vi "SaveImages_Example.vi"() -> ()   [LabVIEW 2019]
doc: "This example shows how to record an image sequence and save all images to files (and an .avi) afterwards.\nIt is a good starting point for writing own applications with file saving\nBut it will not be fail save, i.e. doesnt react on errors, just handles them forward to the end\n\nUsage:\nSelect your required image count you want to record before you start the program.\nOnce started, the camera class will be initialized and images will be recorded automatically.\nWhen acquisition has finished you can read the images by index, crop them using the ROI parameters and select a file path.\nBy clicking save, the images are saved with the selected file format using the current active roi setting.\nThis also finishes the program and will force an exit of the camera class"
uses:
  camera/Camera.lvclass
  pco.recorder/Recorder.lvlib
  <vilib>/picture/picture.llb/Draw 8-Bit Pixmap.vi
  <vilib>/picture/picture.llb/Draw True-Color Pixmap.vi
panel:
  out "colormap(U8)":u32[](array[numeric])
  out "Image(U16)":u16[][](graph)
  in  "Zoom [%]":i32(slide)=26 min=10 max=200 step=5 scale=10.0..200.0
  out "Image":picture
  out "rawImage":u16[][](array[numeric])
  in  "data_format":T1(ring)=enum."Mono16"
  in  "Image Index":u32 max=9
  in  "saveImages":bool
  in  "SavePath":path
  out "Recorded Images":u32
  in  "Quit":bool
  in  "cropY1":u64=2 min=2 max=2048 step=1
  in  "cropX1":u64=2 min=2 max=2048 step=1
  in  "cropY0":u64=1 min=1 max=2047 step=1
  in  "cropX0":u64=1 min=1 max=2047 step=1
  out "Image Height":u16
  out "Image Width":u16
  in  "dwImgCount":u32=10 caption="Required Number of Images" max=4023
  out "Error":errorcluster {"code" format="%x"}
  # "This example shows how to record an image sequence and save all images to files (and an .avi) afterwards.\nIt is a good starting point for writing own applications with file saving\nBut it will not be fail save, i.e. doesnt react on errors, just handles them forward to the end\n\nUsage:\nSelect your required image count you want to record before you start the program.\nOnce started, the camera class will be initialized and images will be recorded automatically.\nWhen acquisition has finished you can read the images by index, crop them using the crop parameters and select a file path.\nBy clicking save, the images are saved with the selected file format using the current active roi setting.\nThis also finishes the program and will force an exit of the camera class"
  # "pco.labview"
  # "Camera Setup"
  # "Recording Control"
  # "Parameters for image readout"
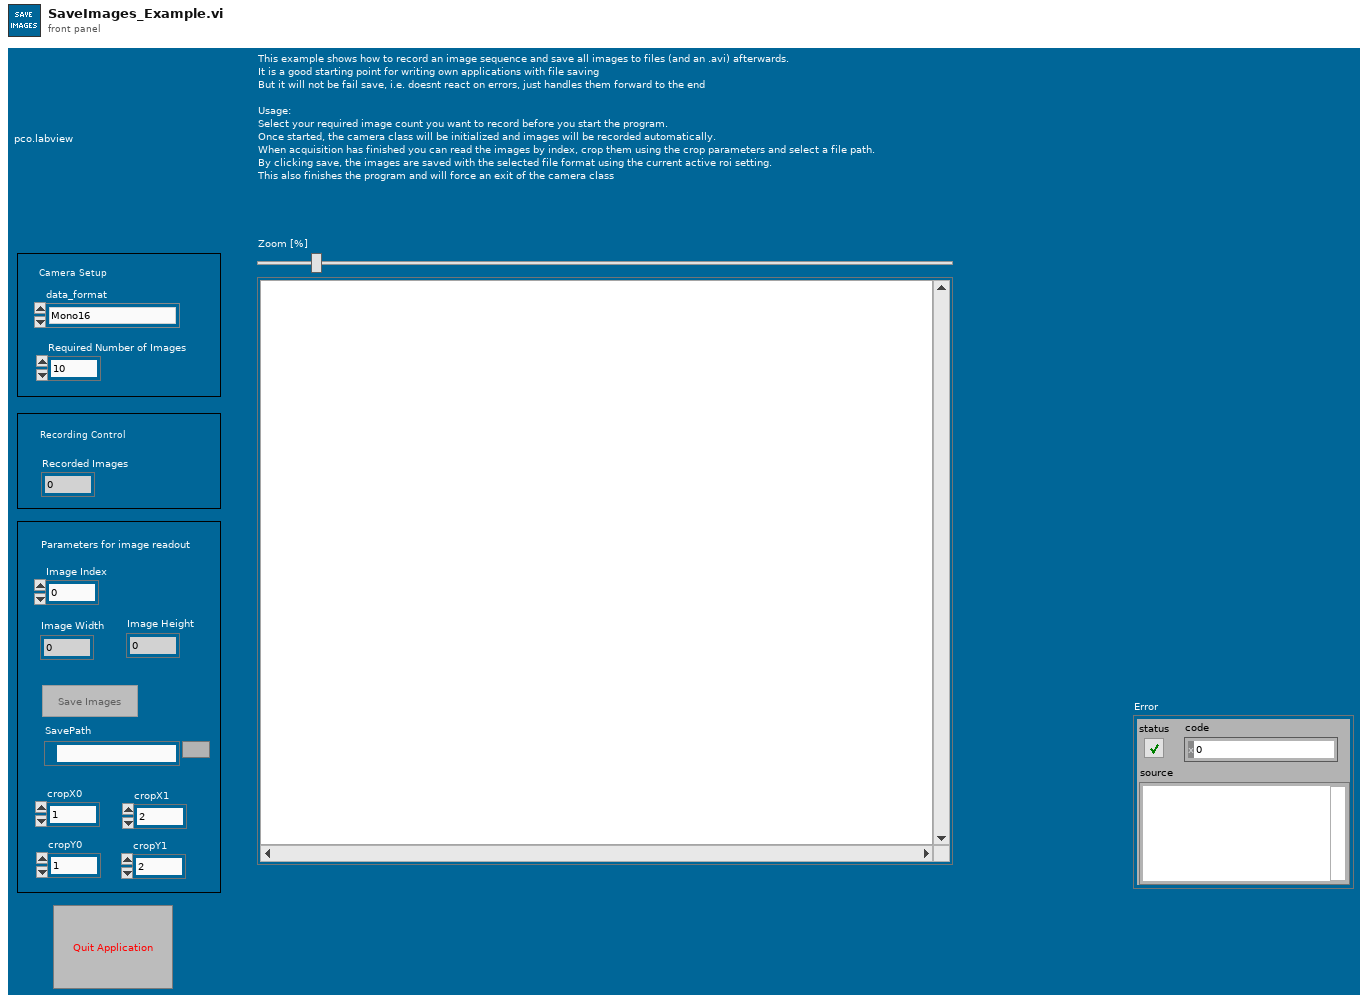
[diagram p1: front panel]
types:
  T1 = enum16{"Undefined", "Mono8", "Mono16", "BGRA8", "RGBA8", "BGRA16", "RGBA16", "CompressedMono8"}
  T2 = enum8{"Enabled", "Disabled", "Disabled and Grayed Out"}
  T3 = enum16{"sequence", "sequence non blocking", "ring buffer", "fifo", "tif", "multitif", "pcoraw", "b16", "dicom", "multidicom", "camram_ring", "camram_segment"}
  T4 = typedef "Camera.lvclass/binning.ctl" = cluster{"vert":u16, "horz":u16, "mode":u16}
  T5 = cluster{"exposure_time_s":dbl, "delay_time_s":dbl, "roi":cluster{"x0":u64, "y0":u64, "x1":u64, "y1":u64}, "timestamp_mode":u16, "pixelrate":u32, "conversion_factor":sgl, "trigger_mode":u16, "acquire_mode":u16, "acquire_sequence_number":u32, "metadata_mode":u16, "noisefilter_mode":u16, "pixel_format":u32, "binning":T4, "auto_exposure":cluster{"region":u16, "min_exposure_s":dbl, "max_exposure_s":dbl}}
  T6 = cluster{"wVersion":u16, "dwIMAGE_COUNTER":u32, "dwIMAGE_TIME_US":u32, "lvTimestamp":timestamp, "bIMAGE_TIME_STATUS":u8, "wEXPOSURE_TIME_BASE":u16, "dwEXPOSURE_TIME":u32, "dwFRAMERATE_MILLIHZ":u32, "sSENSOR_TEMPERATURE":i16, "wIMAGE_SIZE_X":u16, "wIMAGE_SIZE_Y":u16, "bBINNING_X":u8, "bBINNING_Y":u8, "dwSENSOR_READOUT_FREQUENCY":u32, "wSENSOR_CONV_FACTOR":u16, "dwCAMERA_SERIAL_NO":u32, "wCAMERA_TYPE":u16, "bBIT_RESOLUTION":u8, "bSYNC_STATUS":u8, "wDARK_OFFSET":u16, "bTRIGGER_MODE":u8, "bDOUBLE_IMAGE_MODE":u8, "bCAMERA_SYNC_MODE":u8, "bIMAGE_TYPE":u8, "wCOLOR_PATTERN":u16, "wCAMERA_SUBTYPE":u16, "dwEVENT_NUMBER":u32, "wIMAGE_SIZE_X_Offset":u16, "wIMAGE_SIZE_Y_Offset":u16, "bREADOUT_MODE":u8}[]
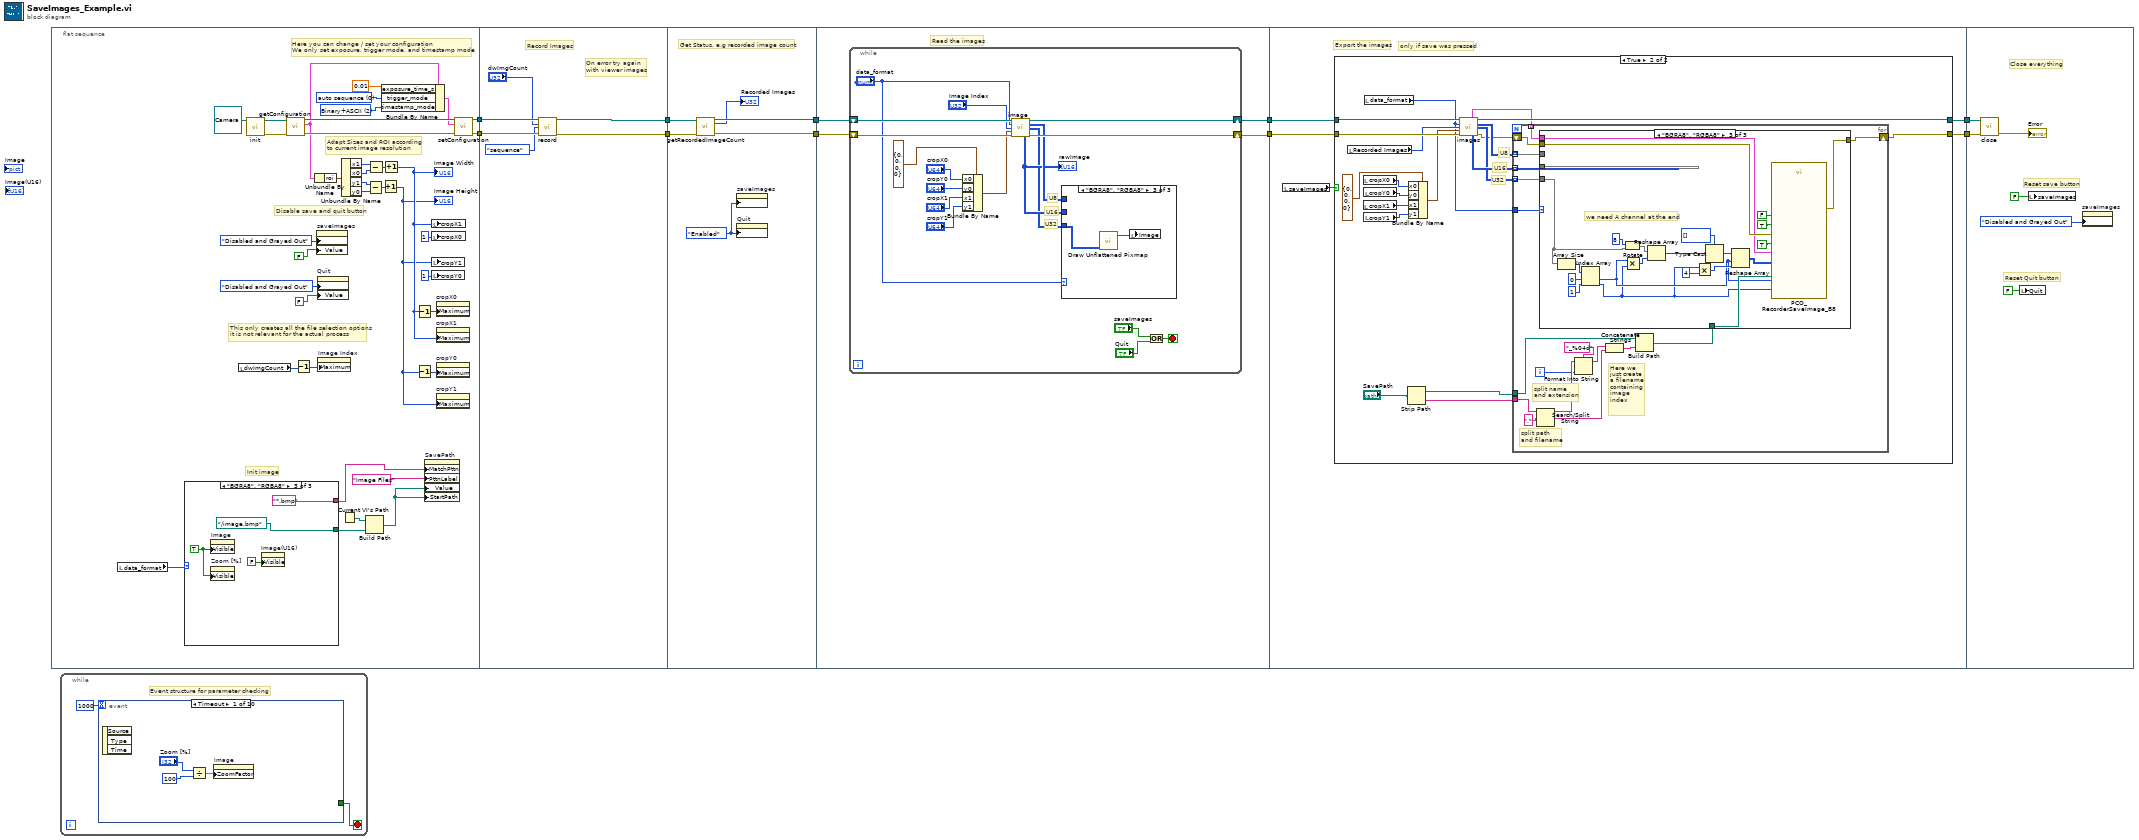
[diagram p0: block diagram]
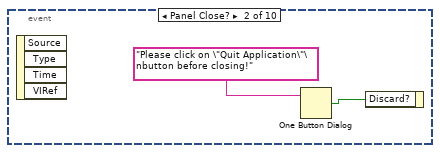
[diagram p2: hidden frame]
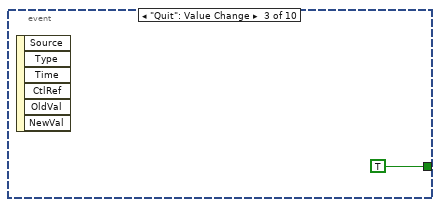
[diagram p3: hidden frame]
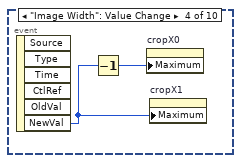
[diagram p4: hidden frame]
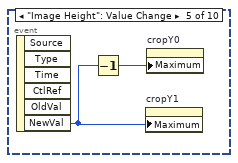
[diagram p5: hidden frame]
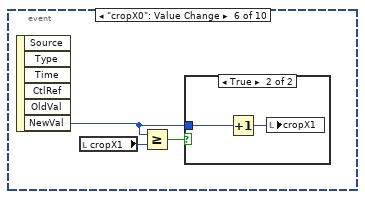
[diagram p6: hidden frame]
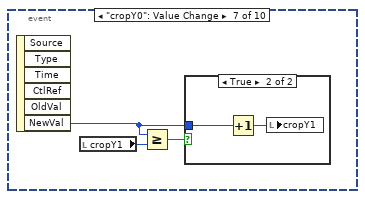
[diagram p8: hidden frame]
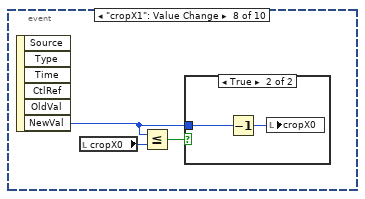
[diagram p10: hidden frame]
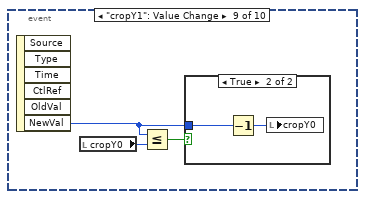
[diagram p12: hidden frame]
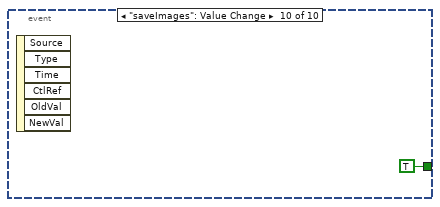
[diagram p14: hidden frame]
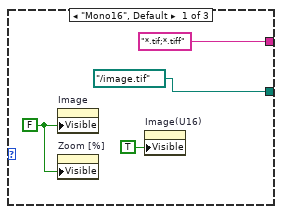
[diagram p15: hidden frame]
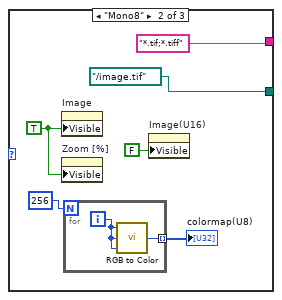
[diagram p16: hidden frame]
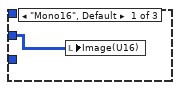
[diagram p17: hidden frame]
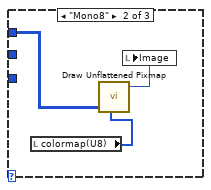
[diagram p18: hidden frame]
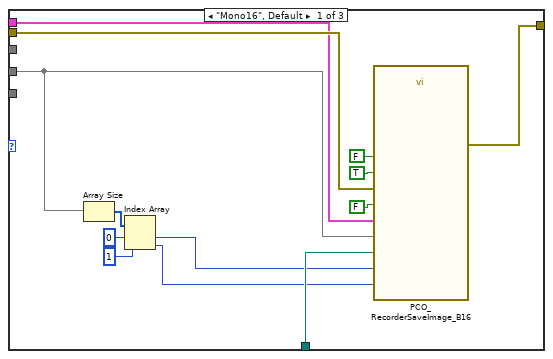
[diagram p20: hidden frame]
diagram:
  n1 = flat-sequence {
    tunnel: [w38] -> w10
    tunnel: [w37] -> w9
    tunnel: w10 -> [w69]
    tunnel: w9 -> [w68]
    tunnel: [w66] -> w8
    tunnel: [w65] -> w7
    tunnel: w8 -> [w75]
    tunnel: w7 -> [w74]
    tunnel: [w73] -> w6
    tunnel: [w72] -> w5
    tunnel: w6 -> [w78]
    tunnel: w5 -> [w79]
    tunnel: [w77] -> w4
    tunnel: [w76] -> w2
    tunnel: w4 -> [w107]
    tunnel: [w106] -> w3
    tunnel: w2 -> [w105]
    tunnel: [w104] -> w1
    tunnel: w3 -> [w201]
    tunnel: w1 -> [w200]
    frame #0 {
      w22 = u16 2 items=["OFF", "Binary", "Binary+ASCII", "ASCII"] ("TimestampMode")
      w44 = u16 0 items=["auto sequence"=0, "software trigger"=1, "external exposure start & software trigger"=2, "external exposure control"=3, "external synchronized"=4, "fast external exposure control"=5, "external CDS control"=6, "slow external exposure control"=7, "external synchronized HDSDI"=258] ("TriggerMode")
      # "Here you can change / set your configuration\nWe only set exposure, trigger mode, and timestamp mode"
      # "Init image"
      # "This only creates all the file selection options\nit is not relevant for the actual process"
      # "Adapt Sizes and ROI according\nto current image resolution"
      # "Disable save and quit button"
      n2 = local read "data_format"() -> (w14:T1)
      n3 = case shown="\"BGRA8\", \"RGBA8\"" w14 {
        tunnel: [path "../image.tif" ("SavePath") path "../image.tif" ("SavePath") path "../image.bmp" ("SavePath")] -> w13
        tunnel: ["*.tif;*.tiff" ("pattern (all files)") "*.tif;*.tiff" ("pattern (all files)") "*.bmp" ("pattern (all files)")] -> w12
        frame "Mono16", Default {
          w50 = FALSE ("Visible")
          n4 = property on="Image" class="Pict"("Visible"=w50) -> ()  [unwired: 2 in, 2 out]
          n5 = property on="Zoom [%]" class="Slide (strict)"("Visible"=w50) -> ()  [unwired: 2 in, 2 out]
          n6 = property on="Image(U16)" class="IntGraph (strict)"("Visible"=TRUE) -> ()  [unwired: 2 in, 2 out]
        }
        frame "Mono8" {
          w56 = TRUE ("Visible")
          n7 = property on="Image" class="Pict"("Visible"=w56) -> ()  [unwired: 2 in, 2 out]
          n8 = property on="Zoom [%]" class="Slide (strict)"("Visible"=w56) -> ()  [unwired: 2 in, 2 out]
          n9 = for {
            N: 256 -> [_]
            tunnel: [w58] -> w55 mode=indexing
            i -> [w59]
            n10 = call <vilib>:"RGB to Color.vi"("B"=w59, "G"=w59, "R"=w59) -> ("Color"=w58:u32)
          }
          "colormap(U8)" <- w55
          n11 = property on="Image(U16)" class="IntGraph (strict)"("Visible"=FALSE) -> ()  [unwired: 2 in, 2 out]
        }
        frame "BGRA8", "RGBA8" {
          w62 = TRUE ("Visible")
          n12 = property on="Image" class="Pict"("Visible"=w62) -> ()  [unwired: 2 in, 2 out]
          n13 = property on="Zoom [%]" class="Slide (strict)"("Visible"=w62) -> ()  [unwired: 2 in, 2 out]
          n14 = property on="Image(U16)" class="IntGraph (strict)"("Visible"=FALSE) -> ()  [unwired: 2 in, 2 out]
        }
      }
      n15 = local read "dwImgCount"() -> (w15:u32)
      n16 = call-dynamic "init.vi"("Camera in"=refnum<class "Camera.lvclass"> refnum ("PCOCamera in")) -> ("Camera out"=w46:refnum<class "Camera.lvclass">, "error out"=w45:errorcluster)  [unwired: 8 in]
      n17 = call-dynamic "getConfiguration.vi"("error in (no error)"=w45, "Camera in"=w46) -> ("error out"=w42:errorcluster, "configuration"=w32:T5, "Camera out"=w43:refnum<class "Camera.lvclass">)  [unwired: 7 in]
      n18 = Decrement(x=w15) -> (x-1=w16:u32)
      n19 = Unbundle By Name(w32) -> ("roi"=w31:cluster{"x0":u64, "y0":u64, "x1":u64, "y1":u64})
      n20 = property on="saveImages" class="Bool (strict)"("DisabledEnum"=T2."Disabled and Grayed Out" ("Disabled"), "Value"=FALSE ("Stop")) -> ()  [unwired: 2 in, 2 out]
      n21 = property on="Quit" class="Bool (strict)"("DisabledEnum"=T2."Disabled and Grayed Out" ("Disabled"), "Value"=FALSE ("Stop")) -> ()  [unwired: 2 in, 2 out]
      n22 = property on="Image Index" class="DigNum (strict)"("Maximum"=w16) -> ()  [unwired: 2 in, 2 out]
      n23 = Current VI's Path() -> (path=w19:path)
      n24 = Unbundle By Name(w31) -> ("x1"=w29:u64, "x0"=w30:u64, "y1"=w27:u64, "y0"=w28:u64)
      n25 = Build Path(base path=w19, name or relative path=w13) -> (appended path=w17:path)
      n26 = Subtract(x=w27, y=w28) -> (x-y=w25:u64)
      n27 = Subtract(x=w29, y=w30) -> (x-y=w26:u64)
      n28 = Bundle By Name(cluster=w32, "exposure_time_s"=0.01, "trigger_mode"=w44, "timestamp_mode"=w22) -> (w41:T5)
      n29 = Increment(x=w25) -> (x+1=w23:u64)
      "Image Height" <- w23
      n30 = Increment(x=w26) -> (x+1=w24:u64)
      "Image Width" <- w24
      n31 = Decrement(x=w24) -> (x-1=w34:u64)
      n32 = Decrement(x=w23) -> (x-1=w33:u64)
      n33 = property on="SavePath" class="Path"("MatchPttn"=w12, "PttnLabel"="Image Files" ("pattern label"), "Value"=w17, "StartPath"=w17) -> ()  [unwired: 2 in, 2 out]
      n34 = local write "cropX1"(w24) -> ()
      n35 = local write "cropX0"(u16 1 ("roiY0")) -> ()
      n36 = local write "cropY1"(w23) -> ()
      n37 = local write "cropY0"(u16 1 ("roiY0")) -> ()
      n38 = property on="cropX0" class="DigNum (strict)"("Maximum"=w34) -> ()  [unwired: 2 in, 2 out]
      n39 = property on="cropX1" class="DigNum (strict)"("Maximum"=w24) -> ()  [unwired: 2 in, 2 out]
      n40 = property on="cropY0" class="DigNum (strict)"("Maximum"=w33) -> ()  [unwired: 2 in, 2 out]
      n41 = property on="cropY1" class="DigNum (strict)"("Maximum"=w23) -> ()  [unwired: 2 in, 2 out]
      n42 = call-dynamic "setConfiguration.vi"("error in (no error)"=w42, "configuration"=w41, "Camera in"=w43) -> ("error out"=w37:errorcluster, "Camera out"=w38:refnum<class "Camera.lvclass">)  [unwired: 7 in]
    }
    frame #1 {
      # "On error try again \nwith viewer images"
      # "Record Images"
      n43 = call-dynamic "record.vi"("Camera in"=w69, "num_images"="dwImgCount", "record_mode"=T3."sequence", "error in (no error)"=w68) -> ("Camera out"=w66:refnum<class "Camera.lvclass">, "error out"=w65:errorcluster)  [unwired: 10 in]
    }
    frame #2 {
      w70 = T2."Enabled" ("Disabled")
      # "Get Status, e.g recorded image count"
      n44 = call-dynamic "getRecordedImageCount.vi"("Camera in"=w75, "error in (no error)"=w74) -> ("Camera out"=w73:refnum<class "Camera.lvclass">, "recorded_image_count"=→"Recorded Images":u32, "error out"=w72:errorcluster)  [unwired: 11 in]
      n45 = property on="saveImages" class="Bool (strict)"("DisabledEnum"=w70) -> ()  [unwired: 2 in, 2 out]
      n46 = property on="Quit" class="Bool (strict)"("DisabledEnum"=w70) -> ()  [unwired: 2 in, 2 out]
    }
    frame #3 {
      # "Read the images"
      n47 = while {
        shift-right: [w95] -> w77
        shift-left: w78 -> [w97]
        shift-right: [w90] -> w76
        shift-left: w79 -> [w96]
        stop <- w88 stop-if-true
        # "U32"
        # "U16"
        # "U8"
        n48 = Bundle By Name(cluster=cluster{"x0":u64, "y0":u64, "x1":u64, "y1":u64} {"x0"=0, "y0"=0, "x1"=0, "y1"=0} ("roi"), "x0"="cropX0", "y0"="cropY0", "x1"="cropX1", "y1"="cropY1") -> (w86:cluster{"x0":u64, "y0":u64, "x1":u64, "y1":u64})
        n49 = call-dynamic "image.vi"("Camera in"=w97, "data_format"="data_format", "image_index"="Image Index", "crop"=w86, "error in (no error)"=w96) -> ("Camera out"=w95:refnum<class "Camera.lvclass">, "image (U8)"=w83:u8[][], "image (U32)"=w81:u32[][], "raw_image (U16)"=w82:u16[][], "error out"=w90:errorcluster)  [unwired: 2 in, 4 out]
        "rawImage" <- w82
        n50 = case shown="\"BGRA8\", \"RGBA8\"" "data_format" {
          tunnel: w81 -> [_ _ w103]
          tunnel: w83 -> [_ w101 _]
          tunnel: w82 -> [w98 _ _]
          frame "Mono16", Default {
            n51 = local write "Image(U16)"(w98) -> ()
          }
          frame "Mono8" {
            n52 = local read "colormap(U8)"() -> (w100:u32[])
            n53 = call-poly <vilib>:"Draw Unflattened Pixmap.vi"("data"=w101, "color table"=w100) -> ("new picture"=w99:picture)  [unwired: 7 in]
            n54 = local write "Image"(w99) -> ()
          }
          frame "BGRA8", "RGBA8" {
            n55 = call-poly <vilib>:"Draw Unflattened Pixmap.vi"("data (RGB format)"=w103) -> ("new picture"=w102:picture)  [unwired: 8 in]
            n56 = local write "Image"(w102) -> ()
          }
        }
        n57 = Or(x="saveImages", y="Quit") -> (x .or. y?=w88:bool)
      }
    }
    frame #4 {
      # "only if save was pressed"
      # "Export the images"
      n58 = local read "saveImages"() -> (w108:bool)
      n59 = case shown="True" w108 {
        tunnel: w107 -> [w110 w129]
        tunnel: [w110 w118] -> w106
        tunnel: w105 -> [w109 w130]
        tunnel: [w109 w112] -> w104
        frame False {
        }
        frame True {
          # "U32"
          # "U16"
          # "U8"
          n60 = local read "Recorded Images"() -> (w122:u32)
          n61 = local read "cropX0"() -> (w127:u64)
          n62 = local read "cropX1"() -> (w125:u64)
          n63 = local read "cropY0"() -> (w126:u64)
          n64 = local read "cropY1"() -> (w124:u64)
          n65 = local read "data_format"() -> (w117:T1)
          n66 = Strip Path(path="SavePath") -> (stripped path=w114:path, name=w115:string)
          n67 = Bundle By Name(cluster=cluster{"x0":u64, "y0":u64, "x1":u64, "y1":u64} {"x0"=0, "y0"=0, "x1"=0, "y1"=0} ("roi"), "x0"=w127, "y0"=w126, "x1"=w125, "y1"=w124) -> (w123:cluster{"x0":u64, "y0":u64, "x1":u64, "y1":u64})
          n68 = call-dynamic "images.vi"("Camera in"=w129, "data_format"=w117, "image_count"=w122, "crop"=w123, "error in (no error)"=w130) -> ("meta_data_list"=w111:T6, "Camera out"=w118:refnum<class "Camera.lvclass">, "image_list (U8)"=w121:u8[][][], "image_list (U32)"=w119:u32[][][], "raw_image_list (U16)"=w120:u16[][][], "error out"=w113:errorcluster)  [unwired: 2 in, 3 out]
          n69 = for {
            tunnel: w121 -> [w147] mode=indexing
            tunnel: w120 -> [w146] mode=indexing
            tunnel: w119 -> [w132] mode=indexing
            tunnel: w117 -> [w138]
            tunnel: w115 -> [w137]
            tunnel: w114 -> [w136]
            shift-right: [w134] -> w112
            shift-left: w113 -> [w135]
            tunnel: w111 -> [w133] mode=indexing
            i -> [w139]
            # "Here we \njust create\na filename\ncontaining\nimage \nindex"
            # "split path \nand filename"
            # "split name \nand extension"
            n70 = Search/Split String(string=w137, search string/char (-)=".") -> (substring before match=w143:string, match + rest of string=w144:string)  [unwired: 1 in, 1 out]
            n71 = Format Into String(format string="_%04d", initial string=w143, w139) -> (resulting string=w145:string)  [unwired: 1 in, 1 out]
            n72 = Concatenate Strings(w145, w144) -> (w140:string)
            n73 = Build Path(base path=w136, name or relative path=w140) -> (appended path=w131:path)
            n74 = case shown="\"BGRA8\", \"RGBA8\"" w138 {
              tunnel: w147 -> [_ w164 _]
              tunnel: w146 -> [w153 _ _]
              tunnel: w135 -> [w157 w170 w192]
              tunnel: [w156 w169 w191] -> w134
              tunnel: w133 -> [w155 w168 w190]
              tunnel: w132 -> [_ _ w177]
              tunnel: w131 -> [w154 w167 w189]
              frame "Mono16", Default {
                n75 = Array Size(array=w153) -> (size(s)=w152:i32[])
                n76 = Index Array(array=w152, index #1=0 ("index"), index #2=1 ("index")) -> (element #1=w150:i32, element #2=w149:i32)
                n77 = call "PCO_RecorderSaveImage_B16.vi"("pImgBuf"=w153, "wWidth"=w149, "wHeight"=w150, "szFilePath"=w154, "error in (no error)"=w157, "isColor"=FALSE, "bIsBitmap"=FALSE, "PCO_METADATA_STRUCT"=w155, "bOverwrite"=TRUE) -> ("error out"=w156:errorcluster)  [unwired: 9 in, 1 out]
              }
              frame "Mono8" {
                n78 = Array Size(array=w164) -> (size(s)=w166:i32[])
                n79 = Index Array(array=w166, index #1=0 ("index"), index #2=1 ("index")) -> (element #1=w163:i32, element #2=w162:i32)
                n80 = call "PCO_RecorderSaveImage_B8.vi"("pImgBuf"=w164, "wWidth"=w162, "wHeight"=w163, "szFilePath"=w167, "error in (no error)"=w170, "isColor"=FALSE, "bIsBitmap"=FALSE, "PCO_METADATA_STRUCT"=w168, "bOverwrite"=TRUE) -> ("error out"=w169:errorcluster)  [unwired: 9 in, 1 out]
              }
              frame "BGRA8", "RGBA8" {
                # "we need A channel at the end"
                n81 = Array Size(array=w177) -> (size(s)=w179:i32[])
                n82 = Index Array(array=w179, index #1=0 ("index"), index #2=1 ("index")) -> (element #1=w176:i32, element #2=w175:i32)
                n83 = Rotate(1:w177, 2:i16 8 ("y")) -> (0:w180:u32[][])
                n84 = Multiply(x=w176, y=w175) -> (x*y=w183:i32)
                n85 = Reshape Array(w180, w183) -> (w182:u32[])
                n86 = Multiply(x=w175, y=u64 4) -> (x*y=w187:u64)
                n87 = Type Cast(type=u8[] [] ("image_list (U32)"), x=w182) -> (*(type *) &x=w188:u8[])
                n88 = Reshape Array(w188, w176, w187) -> (w184:u8[][])
                n89 = call "PCO_RecorderSaveImage_B8.vi"("pImgBuf"=w184, "wWidth"=w175, "wHeight"=w176, "szFilePath"=w189, "error in (no error)"=w192, "isColor"=TRUE, "bIsBitmap"=FALSE, "PCO_METADATA_STRUCT"=w190, "bOverwrite"=TRUE) -> ("error out"=w191:errorcluster)  [unwired: 9 in, 1 out]
              }
            }
          }
        }
      }
    }
    frame #5 {
      # "Reset Quit button"
      # "Close everything"
      # "Reset save button"
      n90 = call-dynamic "close.vi"("error in (no error)"=w200, "Camera in"=w201) -> ("error out"=→"Error":errorcluster)  [unwired: 9 in]
      n91 = local write "Quit"(FALSE ("Stop")) -> ()
      n92 = local write "saveImages"(FALSE ("Stop")) -> ()
      n93 = property on="saveImages" class="Bool (strict)"("DisabledEnum"=T2."Disabled and Grayed Out" ("Disabled")) -> ()  [unwired: 2 in, 2 out]
    }
  }
  n94 = while {
    stop <- w202 stop-if-true
    # "Event structure for parameter checking"
    n95 = event shown="[0] Timeout" {
      selector: _ -> [_ _ _ _ _ _ _ _ _ _]
      dyn-events: _ -> [_ _ _ _ _ _ _ _ _ _]
      timeout: 1000 -> [_ _ _ _ _ _ _ _ _ _]
      tunnel: [_ _ TRUE _ _ _ _ _ _ TRUE] -> w202
      event Timeout {
        n96 = event-data() -> ()  [unwired: 1 in, 3 out]
        n97 = Divide(x="Zoom [%]", y=100 ("Zoom [%]")) -> (x/y=w206:dbl)
        n98 = property on="Image" class="Pict"("ZoomFactor"=w206) -> ()  [unwired: 2 in, 2 out]
      }
      event Panel Close? {
        n99 = event-data() -> ()  [unwired: 1 in, 4 out]
        n100 = One Button Dialog(message="Please click on \"Quit Application\"\nbutton before closing!") -> (true=w207:bool)  [unwired: 1 in]
        n101 = event-data("Discard?"=w207) -> ()  [unwired: 1 in, 1 out]
      }
      event "Quit": Value Change {
        n102 = event-data() -> ()  [unwired: 1 in, 6 out]
      }
      event "Image Width": Value Change {
        n103 = event-data() -> ("NewVal"=w210:u16)  [unwired: 1 in, 5 out]
        n104 = Decrement(x=w210) -> (x-1=w211:u16)
        n105 = property on="cropX0" class="DigNum (strict)"("Maximum"=w211) -> ()  [unwired: 2 in, 2 out]
        n106 = property on="cropX1" class="DigNum (strict)"("Maximum"=w210) -> ()  [unwired: 2 in, 2 out]
      }
      event "Image Height": Value Change {
        n107 = event-data() -> ("NewVal"=w212:u16)  [unwired: 1 in, 5 out]
        n108 = Decrement(x=w212) -> (x-1=w213:u16)
        n109 = property on="cropY1" class="DigNum (strict)"("Maximum"=w212) -> ()  [unwired: 2 in, 2 out]
        n110 = property on="cropY0" class="DigNum (strict)"("Maximum"=w213) -> ()  [unwired: 2 in, 2 out]
      }
      event "cropX0": Value Change {
        n111 = event-data() -> ("NewVal"=w214:u64)  [unwired: 1 in, 5 out]
        n112 = local read "cropX1"() -> (w216:u64)
        n113 = Greater Or Equal?(x=w214, y=w216) -> (x >= y?=w215:bool)
        n114 = case shown="True" w215 {
          tunnel: w214 -> [_ w218]
          frame False {
          }
          frame True {
            n115 = Increment(x=w218) -> (x+1=w217:u64)
            n116 = local write "cropX1"(w217) -> ()
          }
        }
      }
      event "cropY0": Value Change {
        n117 = event-data() -> ("NewVal"=w219:u64)  [unwired: 1 in, 5 out]
        n118 = local read "cropY1"() -> (w221:u64)
        n119 = Greater Or Equal?(x=w219, y=w221) -> (x >= y?=w220:bool)
        n120 = case shown="True" w220 {
          tunnel: w219 -> [_ w223]
          frame False {
          }
          frame True {
            n121 = Increment(x=w223) -> (x+1=w222:u64)
            n122 = local write "cropY1"(w222) -> ()
          }
        }
      }
      event "cropX1": Value Change {
        n123 = event-data() -> ("NewVal"=w224:u64)  [unwired: 1 in, 5 out]
        n124 = local read "cropX0"() -> (w226:u64)
        n125 = Less Or Equal?(x=w224, y=w226) -> (x <= y?=w225:bool)
        n126 = case shown="True" w225 {
          tunnel: w224 -> [_ w228]
          frame False {
          }
          frame True {
            n127 = Decrement(x=w228) -> (x-1=w227:u64)
            n128 = local write "cropX0"(w227) -> ()
          }
        }
      }
      event "cropY1": Value Change {
        n129 = event-data() -> ("NewVal"=w229:u64)  [unwired: 1 in, 5 out]
        n130 = local read "cropY0"() -> (w231:u64)
        n131 = Less Or Equal?(x=w229, y=w231) -> (x <= y?=w230:bool)
        n132 = case shown="True" w230 {
          tunnel: w229 -> [_ w233]
          frame False {
          }
          frame True {
            n133 = Decrement(x=w233) -> (x-1=w232:u64)
            n134 = local write "cropY0"(w232) -> ()
          }
        }
      }
      event "saveImages": Value Change {
        n135 = event-data() -> ()  [unwired: 1 in, 6 out]
      }
    }
  }
